vi "Basic Test SubVI.vi"() -> ()   [LabVIEW 2023]
panel:
  in  "Numeric":dbl
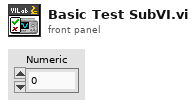
[diagram p1: front panel]
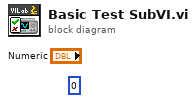
[diagram p0: block diagram]
diagram:
  (unwired) 0
